vi "Mem32.vi"(4 "Phi1":bool, 6 "Phi0":bool, 11 "Data In":bool) -> (3 "Data Out":bool)   [LabVIEW 2012]
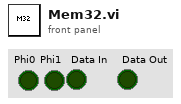
[diagram p1: front panel]
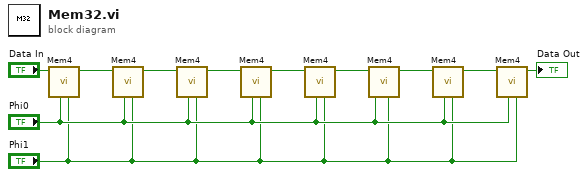
[diagram p0: block diagram]
diagram:
  n1 = call "Mem4.vi"("Phi1"="Phi1", "Phi0"="Phi0", "Data In"="Data In") -> ("Data Out"=w8:bool)  [unwired: 8 in]
  n2 = call "Mem4.vi"("Phi1"="Phi1", "Phi0"="Phi0", "Data In"=w8) -> ("Data Out"=w7:bool)  [unwired: 8 in]
  n3 = call "Mem4.vi"("Phi1"="Phi1", "Phi0"="Phi0", "Data In"=w7) -> ("Data Out"=w6:bool)  [unwired: 8 in]
  n4 = call "Mem4.vi"("Phi1"="Phi1", "Phi0"="Phi0", "Data In"=w6) -> ("Data Out"=w5:bool)  [unwired: 8 in]
  n5 = call "Mem4.vi"("Phi1"="Phi1", "Phi0"="Phi0", "Data In"=w5) -> ("Data Out"=w4:bool)  [unwired: 8 in]
  n6 = call "Mem4.vi"("Phi1"="Phi1", "Phi0"="Phi0", "Data In"=w4) -> ("Data Out"=w3:bool)  [unwired: 8 in]
  n7 = call "Mem4.vi"("Phi1"="Phi1", "Phi0"="Phi0", "Data In"=w3) -> ("Data Out"=w2:bool)  [unwired: 8 in]
  n8 = call "Mem4.vi"("Phi1"="Phi1", "Phi0"="Phi0", "Data In"=w2) -> ("Data Out"=→"Data Out":bool)  [unwired: 8 in]
